vi "TDMS_test.vi"() -> ()   [LabVIEW 2016]
panel:
  out "Full time, ms":u32
  out "time to run 1 cycle, ms":dbl
  in  "file path":path
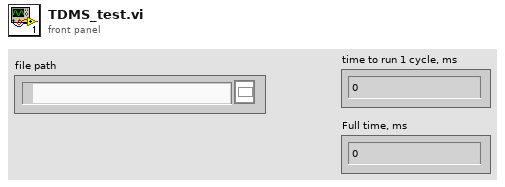
[diagram p1: front panel]
types:
  T1 = enum16{"open", "open or create", "create or replace", "create", "open (read-only)"}
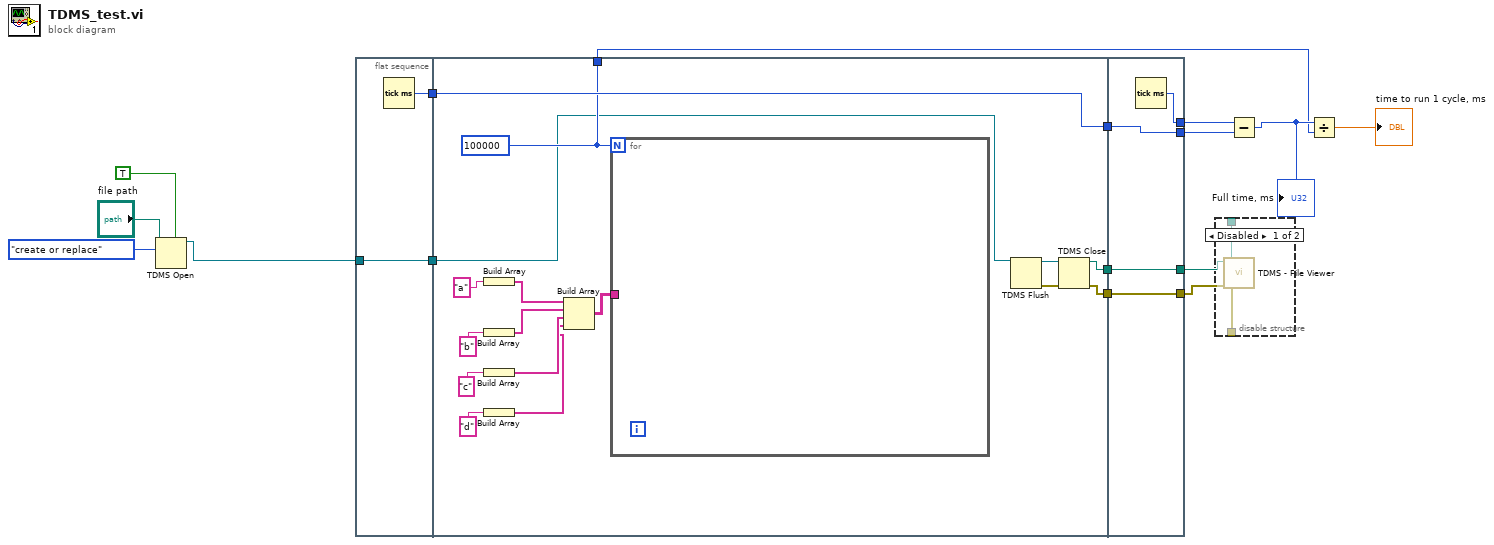
[diagram p0: block diagram]
diagram:
  n1 = TDMS Open(5:TRUE ("create index file? (T)"), 10:T1."create or replace" ("operation (0:open)"), 11:"file path") -> (3:w14:refnum<k34>)  [unwired: 4 in, 1 out]
  n2 = flat-sequence {
    tunnel: w14 -> [w18]
    tunnel: [w18] -> w13
    tunnel: [w17] -> w7
    tunnel: w13 -> [w19]
    tunnel: [w32] -> w12
    tunnel: [w31] -> w11
    tunnel: [w30] -> w8
    tunnel: w7 -> [w30]
    tunnel: [w29] -> w5
    tunnel: [w37] -> w2
    tunnel: [w38] -> w3
    tunnel: w12 -> [w38]
    tunnel: w11 -> [w37]
    tunnel: [w36] -> w10
    tunnel: [w35] -> w9
    tunnel: w8 -> [w35]
    frame #0 {
      n3 = Tick Count (ms)() -> (millisecond timer value=w17:u32)
    }
    frame #1 {
      w29 = 100000
      n4 = Build Array("a") -> (w28:string[])
      n5 = Build Array("b") -> (w26:string[])
      n6 = Build Array("c") -> (w25:string[])
      n7 = Build Array("d") -> (w24:string[])
      n8 = Build Array(w28, w26, w25, w24) -> (w27:string[][])
      n9 = for {
        N: w29 -> [_]
        tunnel: w27 -> [_]
      }
      n10 = TDMS Flush(7:w19) -> (0:w34:errorcluster, 3:w33:refnum<k34>)  [unwired: 1 in]
      n11 = TDMS Close(8:w34, 11:w33) -> (0:w31:errorcluster, 3:w32:path)
    }
    frame #2 {
      n12 = Tick Count (ms)() -> (millisecond timer value=w36:u32)
    }
  }
  n13 = disable-structure shown="Disabled" {
    disable-tunnel: w3 -> [w40 _]
    disable-tunnel: w2 -> [w39 _]
    frame Disabled {
      n14 = call <vilib>:"TDMS - File Viewer.vi"("error in (no error)"=w39, "file path"=w40) -> ()  [unwired: 4 in, 2 out]
    }
    frame Enabled {
    }
  }
  n15 = Subtract(x=w10, y=w9) -> (x-y=w6:u32)
  "Full time, ms" <- w6
  n16 = Divide(x=w6, y=w5) -> (x/y=→"time to run 1 cycle, ms":dbl)
